vi "Open from SFTP.vi"(8 "Error In":errorcluster, 10 "Remote Path":string, 11 "SFTP":refnum<class "SFTP.lvclass">) -> (0 "Error Out":errorcluster, 3 "SFTP Directory":refnum<class "SFTP Directory.lvclass">)   [LabVIEW 2021, in "Field_RnD_Services_LIBSSH2_Toolkit.lvlib" / "SFTP Directory.lvclass"]
doc: "Creates a new SFTP Directory object from a SFTP object."
uses:
  220524-VNA RP FLAT.llb/SFTP Directory.lvclass
  220524-VNA RP FLAT.llb/SFTP.lvclass
  220524-VNA RP FLAT.llb/SFTP Directory.lvclass/SFTP Directory.ctl
  220524-VNA RP FLAT.llb/Field_RnD_Services_LIBSSH2_Toolkit.lvlib
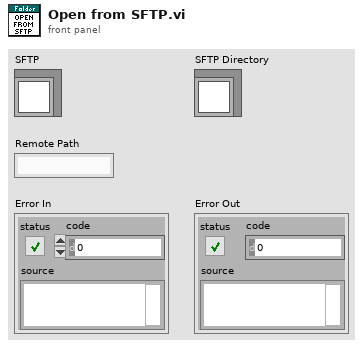
[diagram p1: front panel]
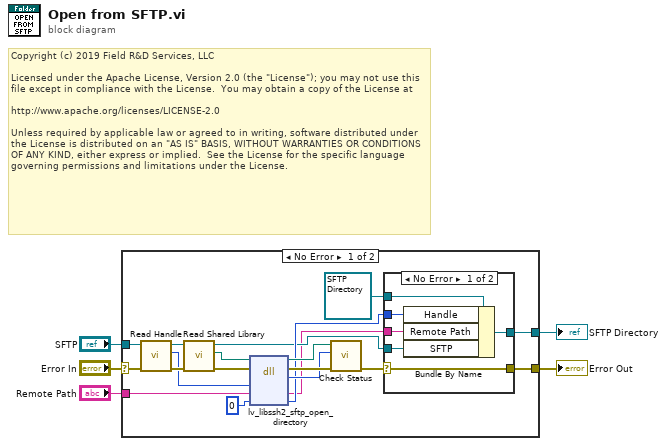
[diagram p0: block diagram]
diagram:
  # "Copyright (c) 2019 Field R&D Services, LLC\n\nLicensed under the Apache License, Version 2.0 (the \"License\"); you may not use this file except in compliance with the License.  You may obtain a copy of the License at\n\nhttp://www.apache.org/licenses/LICENSE-2.0\n\nUnless required by applicable law or agreed to in writing, software distributed under the License is distributed on an \"AS IS\" BASIS, WITHOUT WARRANTIES OR CONDITIONS OF ANY KIND, either express or implied.  See the License for the specific language governing permissions and limitations under the License."
  n1 = case shown="No Error" "Error In" {
    selector: "Error In" -> [w18 w33]
    tunnel: [w7 w33] -> w4
    tunnel: "SFTP" -> [w19 _]
    tunnel: "Remote Path" -> [w24 _]
    tunnel: [w10 _] -> w1
    frame No Error {
      n2 = call "Read Handle.vi"("Error In"=w18, "SFTP In"=w19) -> ("Erorr Out"=w16:errorcluster, "Handle"=w14:u64, "SFTP Out"=w17:refnum<class "SFTP.lvclass">)  [unwired: 7 in]
      n3 = call "Read Shared Library.vi"("Error In"=w16, "SFTP In"=w17) -> ("Erorr Out"=w13:errorcluster, "libssh2lv Shared Library"=w15:path, "SFTP Out"=w9:refnum<class "SFTP.lvclass">)  [unwired: 7 in]
      n4 = dll-call lib="lv-libssh2.*" fn="lv_libssh2_sftp_open_directory"(path in=w15, error in=w13, "sftp"=w14, "path"=w24, "handle"=u64 0) -> (path out=w23:path, error out=w22:errorcluster, "status"=w21:i32, "path"=w6:string, "handle"=w11:u64)  [unwired: 2 in]
      n5 = call "Check Status.vi"("Error In"=w22, "Status"=w21, "libssh2lv Shared Library In"=w23) -> ("Error Out"=w8:errorcluster)  [unwired: 7 in, 1 out]
      n6 = case shown="No Error" w8 {
        selector: w8 -> [w26 w32]
        tunnel: refnum<class "SFTP Directory.lvclass"> refnum ("Toolkit.lvlib:SFTP Directory.lvclass") -> [w30 w31]
        tunnel: w11 -> [w29 _]
        tunnel: [w28 w31] -> w10
        tunnel: w9 -> [w27 _]
        tunnel: [w26 w32] -> w7
        tunnel: w6 -> [w25 _]
        frame No Error {
          n7 = Bundle By Name(cluster=w30, "Handle"=w29, "Remote Path"=w25, "SFTP"=w27) -> (w28:refnum<class "SFTP Directory.lvclass">)
        }
        frame Error {
        }
      }
    }
    frame Error {
    }
  }
  "Error Out" <- w4
  "SFTP Directory" <- w1
